vi "AutoTurn.vi"(8 "error in (no error)":errorcluster, 9 "Setpoint":dbl, 10 "GyroDevRef":T1={"DevStatus"={"status"=FALSE, "code"=0, "source"=""}, "Analog Channel"=enum."AI 0", "Gain (VoltsPerDegree/Second)"=0.0, "Gyro Type"=enum."Analog", "Handle"=0, "SPI Bus"=enum."Invalid", "Device Found"=FALSE, "Sample Rate"=1.0, "Calibrate On Open"=FALSE, "Offset"=0.0} {"Sample Rate" min=0.25 max=100.0 step=0.25}, 11 "RobotDriveDevRef":T4={"DevStatus"={"status"=FALSE, "code"=0, "source"=""}, "Motors[]"=[], "Square Inputs"=FALSE, "Max Output"=1.0}) -> (0 "error out":errorcluster)   [LabVIEW 2017]
uses:
  <vilib>/Rock Robotics/WPI/RobotDrive/WPI_RobotDriveDevRef.ctl
  <vilib>/Rock Robotics/WPI/MotorControl/WPI_MotorControlDeviceRef.ctl
  <vilib>/Rock Robotics/WPI/MotorControl/WPI_MotorControlType.ctl
  <vilib>/Rock Robotics/SystemInterfaces/DIO/FPGA_DIOPWMChannel.ctl
  <vilib>/Rock Robotics/WPI/PWM/WPI_PWMDeadband.ctl
  <vilib>/Rock Robotics/SystemInterfaces/DIO/FPGA_DIOChannel.ctl
  <vilib>/Rock Robotics/WPI/Gyro/WPI_GyroDevRef.ctl
  <vilib>/Rock Robotics/SystemInterfaces/AI/FPGA_AIChannel.ctl
  <vilib>/Rock Robotics/SystemInterfaces/spilib/spi_bus.ctl
  <vilib>/Rock Robotics/Network Tables/NT Write Number.vi
  <vilib>/Rock Robotics/WPI/RobotDrive/WPI_RobotDriveArcadeDrive_Standard(NoSaturation).vi
panel:
  # "Analog"
  # "XRS"
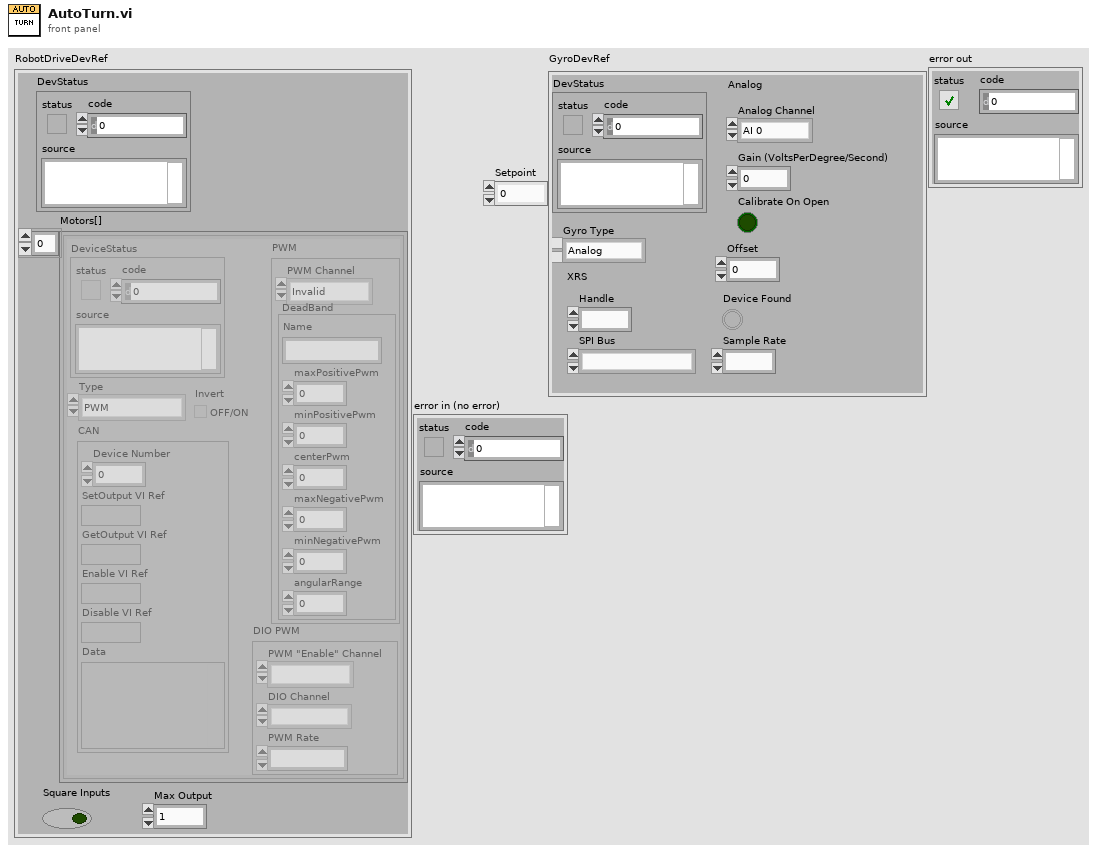
[diagram p1: front panel]
types:
  T1 = typedef "WPI_GyroDevRef.ctl" = cluster{"DevStatus":errorcluster, "Analog Channel":T2, "Gain (VoltsPerDegree/Second)":dbl, "Gyro Type":enum16{"Analog", "XRS450"}, "Handle":i32, "SPI Bus":T3, "Device Found":bool, "Sample Rate":dbl, "Calibrate On Open":bool, "Offset":dbl}
  T2 = typedef "FPGA_AIChannel.ctl" = enum8{"AI 0", "AI 1", "AI 2", "AI 3", "AI MXP 0", "AI MXP 1", "AI MXP 2", "AI MXP 3", "Invalid"}
  T3 = typedef "spi_bus.ctl" = enum16{"SPI On-Board, CS0", "SPI On-Board, CS1", "SPI On-Board, CS2", "SPI On-Board, CS3", "SPI MXP", "Invalid"}
  T4 = typedef "WPI_RobotDriveDevRef.ctl" = cluster{"DevStatus":errorcluster, "Motors[]":T5[], "Square Inputs":bool, "Max Output":dbl}
  T5 = typedef "WPI_MotorControlDeviceRef.ctl" = cluster{"DeviceStatus":errorcluster, "Type":T6, "PWM":cluster{"PWM Channel":T7, "DeadBand":T8}, "CAN":cluster{"Device Number":u8, "SetOutput VI Ref":variant, "GetOutput VI Ref":variant, "Enable VI Ref":variant, "Disable VI Ref":variant, "Data":variant}, "Invert":bool, "DIO PWM":cluster{"PWM \"Enable\" Channel":T7, "DIOChannel":T9, "PWM Rate":dbl}}
  T6 = typedef "WPI_MotorControlType.ctl" = enum16{"PWM", "CAN", "DIO PWM"}
  T7 = typedef "FPGA_DIOPWMChannel.ctl" = enum8{"PWM 0", "PWM 1", "PWM 2", "PWM 3", "PWM 4", "PWM 5", "PWM 6", "PWM 7", "PWM 8", "PWM 9", "PWM MXP 0", "PWM MXP 1", "PWM MXP 2", "PWM MXP 3", "PWM MXP 4", "PWM MXP 5", "PWM MXP 6", "PWM MXP 7", "PWM MXP 8", "PWM MXP 9", "Invalid"}
  T8 = typedef "WPI_PWMDeadband.ctl" = cluster{"Name":string, "maxPositivePwm":i32, "minPositivePwm":i32, "centerPwm":i32, "maxNegativePwm":i32, "minNegativePwm":i32, "angularRange":u16}
  T9 = typedef "FPGA_DIOChannel.ctl" = enum8{"DIO 0", "DIO 1", "DIO 2", "DIO 3", "DIO 4", "DIO 5", "DIO 6", "DIO 7", "DIO 8", "DIO 9", "DIO MXP 0", "DIO MXP 1", "DIO MXP 2", "DIO MXP 3", "DIO MXP 4", "DIO MXP 5", "DIO MXP 6", "DIO MXP 7", "DIO MXP 8", "DIO MXP 9", "DIO MXP 10", "DIO MXP 11", "DIO MXP 12", "DIO MXP 13", "DIO MXP 14", "DIO MXP 15", "SPI Port CS1", "SPI Port CS2", "SPI Port CS3", "SPI Port MISO", "SPI Port MOSI", "Invalid"}
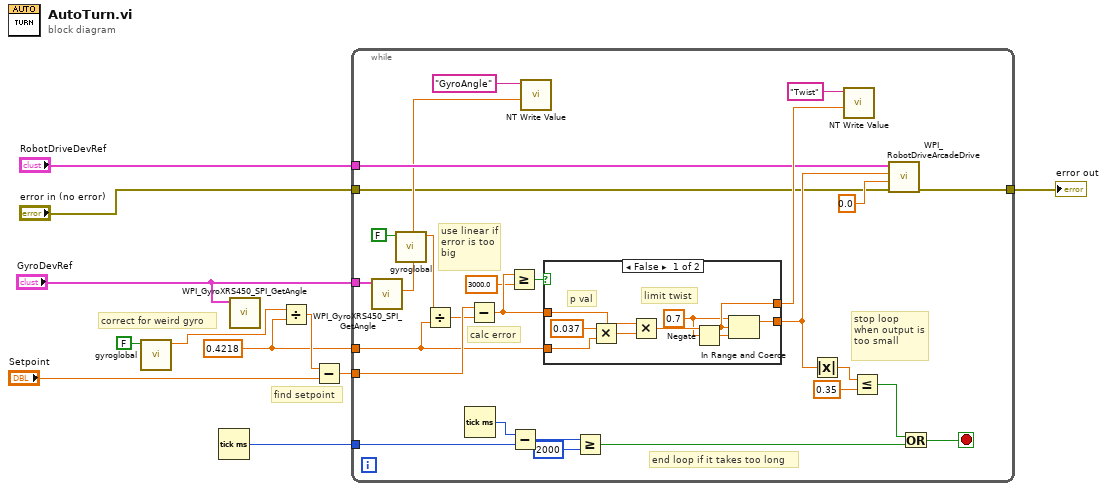
[diagram p0: block diagram]
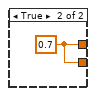
[diagram p2: hidden frame]
diagram:
  w9 = 0.4218 ("y")
  # "find setpoint"
  # "correct for weird gyro"
  n1 = call "gyroglobal.vi"("Set(T)/Get(F)"=FALSE) -> ("Angle"=w2:dbl)  [unwired: 9 in, 1 out]
  n2 = Tick Count (ms)() -> (millisecond timer value=w3:u32)
  n3 = call <vilib>:"WPI_GyroXRS450_SPI_GetAngle.vi"("GyroDevRef"="GyroDevRef") -> ()  [unwired: 6 in, 5 out]
  n4 = Divide(x=w2, y=w9) -> (x/y=w10:dbl)
  n5 = Subtract(x=w10, y="Setpoint") -> (x-y=w11:dbl)
  n6 = while {
    tunnel: "RobotDriveDevRef" -> [w34]
    tunnel: "GyroDevRef" -> [w35]
    tunnel: w11 -> [w33]
    tunnel: w9 -> [w26]
    tunnel: "error in (no error)" -> [w21]
    tunnel: [w20] -> w4
    tunnel: w3 -> [w18]
    stop <- w15 stop-if-true
    # "end loop if it takes too long"
    # "stop loop when output is too small"
    # "use linear if error is too big"
    # "calc error"
    n7 = call <vilib>:"WPI_GyroXRS450_SPI_GetAngle.vi"("GyroDevRef"=w35) -> ("Angle"=w31:dbl)  [unwired: 6 in, 4 out]
    n8 = call "gyroglobal.vi"("Set(T)/Get(F)"=FALSE) -> ("Angle"=w12:dbl)  [unwired: 9 in, 1 out]
    n9 = Divide(x=w12, y=w26) -> (x/y=w27:dbl)
    n10 = Tick Count (ms)() -> (millisecond timer value=w19:u32)
    n11 = Subtract(x=w33, y=w27) -> (x-y=w25:dbl)
    n12 = Greater Or Equal?(x=w25, y=3000.0) -> (x >= y?=w23:bool)
    n13 = Subtract(x=w19, y=w18) -> (x-y=w17:u32)
    n14 = call-poly <vilib>:"NT Write Value.vi"("Numeric"=w31, "Name"="GyroAngle") -> ()  [unwired: 9 in, 1 out]
    n15 = case shown="False" w23 {
      tunnel: [w46 w47] -> w22
      tunnel: [w45 w47] -> w37
      tunnel: w25 -> [w44 _]
      tunnel: w26 -> [w42 _]
      frame False {
        w39 = 0.7 ("upper limit")
        # "limit twist"
        # "p val"
        n16 = Multiply(x=0.037, y=w42) -> (x*y=w43:dbl)
        n17 = Multiply(x=w44, y=w43) -> (x*y=w45:dbl)
        n18 = Negate(x=w39) -> (-x=w40:dbl)
        n19 = In Range and Coerce(upper limit=w39, x=w45, lower limit=w40) -> (coerced(x)=w46:dbl)  [unwired: 1 out]
      }
      frame True {
        w47 = 0.7
      }
    }
    n20 = Greater Or Equal?(x=w17, y=u32 2000) -> (x >= y?=w14:bool)
    n21 = Absolute Value(x=w22) -> (abs(x)=w30:dbl)
    n22 = call-poly <vilib>:"NT Write Value.vi"("Numeric"=w37, "Name"="Twist") -> ()  [unwired: 9 in, 1 out]
    n23 = Less Or Equal?(x=w30, y=0.35) -> (x <= y?=w28:bool)
    n24 = call-poly <vilib>:"WPI_RobotDriveArcadeDrive.vi"("error in (no error)"=w21, "Y axis value"=0.0, "X axis value"=w22, "RobotDriveDevRef"=w34) -> ("error out"=w20:errorcluster)  [unwired: 5 in, 2 out]
    n25 = Or(x=w28, y=w14) -> (x .or. y?=w15:bool)
  }
  "error out" <- w4
